vi "Build.vi"(8 "error in (no error)":errorcluster, 10 "Pizza":refnum<class "Pizza(Product).lvclass">, 11 "HawaiianPizzaBuilder in":refnum<class "HawaiianPizzaBuilder.lvclass">) -> (0 "error out":errorcluster, 2 "Pizza out":refnum<class "Pizza(Product).lvclass">, 3 "HawaiianPizzaBuilder out":refnum<class "HawaiianPizzaBuilder.lvclass">)   [LabVIEW 2014, in "HawaiianPizzaBuilder.lvclass"]
uses:
  HawaiianPizzaBuilder.lvclass
  Pizza(Product)/Pizza(Product).lvclass
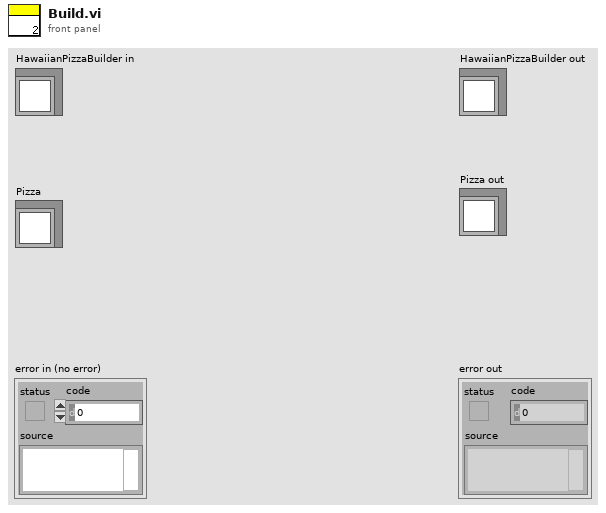
[diagram p1: front panel]
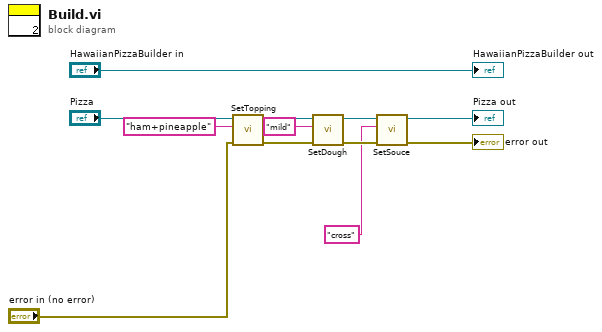
[diagram p0: block diagram]
diagram:
  n1 = call "SetTopping.vi"("error in (no error)"="error in (no error)", "Topping"="ham+pineapple", "object in"="Pizza") -> ("error out"=w6:errorcluster, "object out"=w10:refnum<class "Pizza(Product).lvclass">)  [unwired: 7 in]
  n2 = call "SetDough.vi"("error in (no error)"=w6, "Dough"="mild", "object in"=w10) -> ("error out"=w5:errorcluster, "object out"=w9:refnum<class "Pizza(Product).lvclass">)  [unwired: 7 in]
  n3 = call "SetSouce.vi"("error in (no error)"=w5, "Souce"="cross", "object in"=w9) -> ("error out"=→"error out":errorcluster, "object out"=→"Pizza out":refnum<class "Pizza(Product).lvclass">)  [unwired: 7 in]
  "HawaiianPizzaBuilder out" <- "HawaiianPizzaBuilder in"
